vi "Capture Peak Index (SubVI).vi"(9 "Peak Index":u16, 10 "Dip Valid?":bool, 11 "Peak Count":u16) -> (3 "Peak Index Array":u16[](array[numeric]))   [LabVIEW 2015]
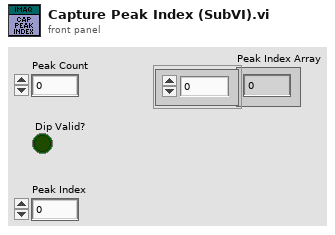
[diagram p1: front panel]
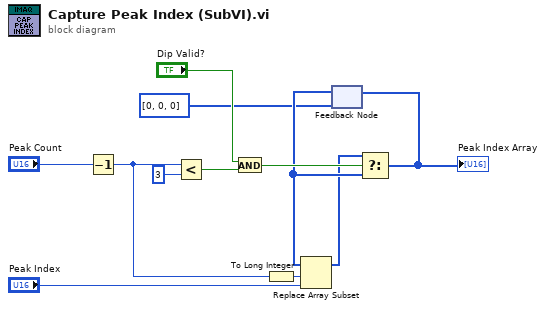
[diagram p0: block diagram]
diagram:
  n1 = Decrement(x="Peak Count") -> (x-1=w8:u16)
  n2 = Less?(x=w8, y=u16 3) -> (x < y?=w7:bool)
  n3 = And(x="Dip Valid?", y=w7) -> (x .and. y?=w10:bool)
  n4 = To Long Integer(number=w8) -> (32bit integer=w2:i32)
  n5 = feedback #1(u16[] [0, 0, 0]) -> (w6:u16[])
  n6 = Replace Array Subset(array=w6, new element="Peak Index", index=w2) -> (w4:u16[])
  n7 = Select(t=w4, s=w10, f=w6) -> (s? t:f=w12:u16[])
  "Peak Index Array" <- w12
  n8 = feedback-in #1(w12) -> ()
